vi "Activate dub.vi"(7 "DO Task":refnum<k21>, 8 "error constant":errorcluster, 11 "DO":T1(array[cluster])=[{"CDT"=-150.0, "Position"=TRUE, "Component ID"="F_EPV_131"}, {"CDT"=-150.0, "Position"=TRUE, "Component ID"="F_EPV_131"}, {"CDT"=-135.0, "Position"=FALSE, "Component ID"="F_EPV_132"}, {"CDT"=-120.0, "Position"=FALSE, "Component ID"="F_EPV_131"}, {"CDT"=-20.0, "Position"=TRUE, "Component ID"="F_EPV_136"}, {"CDT"=-10.0, "Position"=FALSE, "Component ID"="F_EPV_136"}]) -> (0 "error out":errorcluster, 3 "Abort":bool)   [LabVIEW 2022 SP3]
uses:
  RT Controls/DO FGV.ctl
  <vilib>/DAQmx/write.llb/DAQmx Write (Digital 1D Bool NChan 1Samp 1Line).vi
  RT Sub VI's/RT Global.vi
  <vilib>/DAQmx/miscellaneous.llb/DAQmx Fill In Error Info.vi
panel:
  out "Launch Time":timestamp
  out "DO value":bool[](array[boolean])
  out "Status":string
  out "x-y":dbl
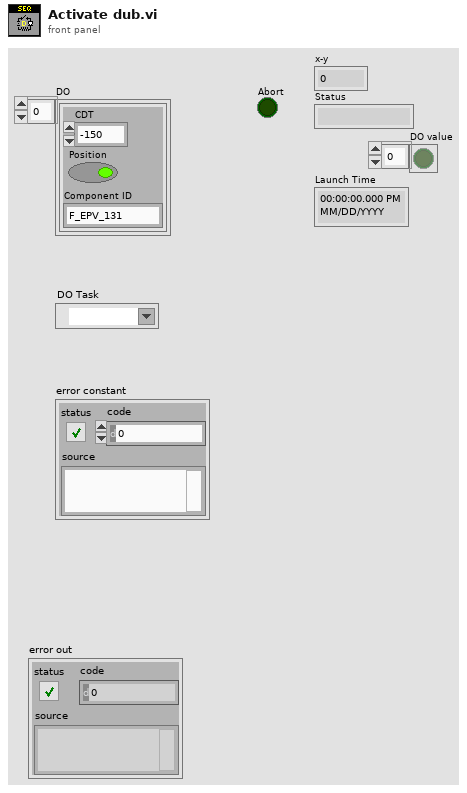
[diagram p1: front panel]
types:
  T1 = cluster{"CDT":dbl, "Position":bool, "Component ID":string}[]
  T2 = cluster{"AO":cluster{"CDT":dbl, "Range":dbl, "Component ID":string}[], "DO":cluster{"CDT":dbl, "Position":bool, "Component ID":string}[], "Launch Time":timestamp}
  T3 = typedef "DO FGV.ctl" = enum16{"Read", "Write", "Start time", "init", "Read only"}
  T4 = cluster{"CDT":dbl, "Position":bool, "Component ID":string}
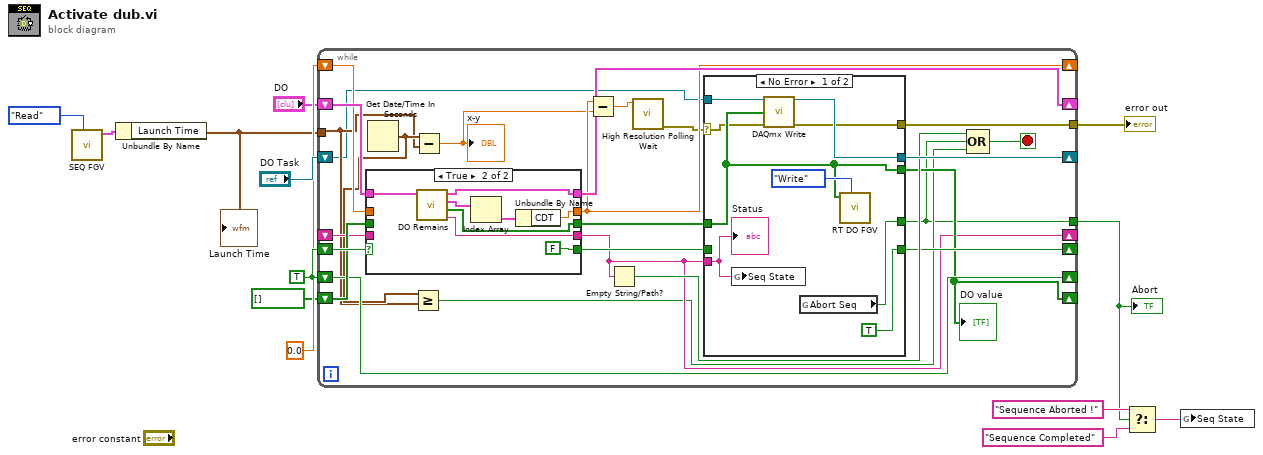
[diagram p0: block diagram]
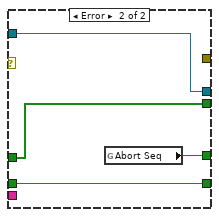
[diagram p2: hidden frame]
diagram:
  w13 = TRUE
  n1 = call "SEQ FGV.vi"("Enum"=enum16{"Read", "Write"}."Read") -> ("Seq data out"=w10:T2)  [unwired: 9 in, 1 out]
  n2 = Unbundle By Name(w10) -> ("Launch Time"=w1:timestamp)
  "Launch Time" <- w1
  n3 = while {
    shift-right: [w30] -> _
    shift-left: "DO" -> [w38]
    shift-right: [w27] -> _
    shift-left: w13 -> [w37]
    shift-right: [w26] -> _
    shift-left: bool[] [] ("DO value") -> [w36]
    shift-right: [w20] -> _
    shift-left: 0.0 ("CDT") -> [w35]
    shift-right: [w33] -> _
    shift-left: w13 -> [w33]
    shift-right: [w32] -> _
    shift-left: "DO Task" -> [w15]
    tunnel: [w16] -> w4
    tunnel: w1 -> [w22]
    shift-right: [w24] -> _
    shift-left: _ -> [w25]
    tunnel: [w17] -> w3
    stop <- w31 stop-if-true
    n4 = case shown="True" w37 {
      selector: w37 -> [w53 _]
      tunnel: w38 -> [w54 w64]
      tunnel: [w54 w59] -> w30
      tunnel: [w56 w61] -> w34
      tunnel: w36 -> [w56 _]
      tunnel: [w55 w60] -> w20
      tunnel: w35 -> [w55 _]
      tunnel: [w53 FALSE] -> w28
      tunnel: [w52 w57] -> w24
      tunnel: w25 -> [w52 _]
      frame False {
      }
      frame True {
        n5 = call "DO Remains.vi"("Array"=w64) -> ("Status"=w57:string, "DO value"=w61:bool[], "Same DO"=w63:T1, "Remains"=w59:T1)  [unwired: 7 in]
        n6 = Index Array(array=w63) -> (element=w62:T4)  [unwired: 1 in]
        n7 = Unbundle By Name(w62) -> ("CDT"=w60:dbl)
      }
    }
    n8 = Get Date/Time In Seconds() -> (seconds since 1Jan1904=w23:timestamp)
    n9 = Greater Or Equal?(x=w23, y=w22) -> (x >= y?=w21:bool)
    n10 = Subtract(x=w23, y=w22) -> (x-y=w19:dbl)
    "x-y" <- w19
    n11 = Subtract(x=w20, y=w19) -> (x-y=w14:dbl)
    n12 = Empty String/Path?(string/path=w24) -> (empty?=w29:bool)
    n13 = call <vilib>:"High Resolution Polling Wait.vi"("seconds to wait"=w14) -> ("error out"=w18:errorcluster)  [unwired: 10 in]
    n14 = case shown="No Error" w18 {
      selector: w18 -> [w40 _]
      tunnel: w34 -> [w41 w51]
      tunnel: [w41 w51] -> w26
      tunnel: w15 -> [w47 w50]
      tunnel: [w46 w50] -> w32
      tunnel: [w45 _] -> w17
      tunnel: w28 -> [_ w49]
      tunnel: [TRUE w49] -> w27
      tunnel: w24 -> [w43 _]
      tunnel: [w39 w48] -> w16
      frame No Error {
        n15 = global write "RT Global.vi" "Seq State"(w43) -> ()
        n16 = call-poly <vilib>:"DAQmx Write.vi"("task/channels in"=w47, "data"=w41, "error in"=w40) -> ("task out"=w46:refnum<k21>, "error out"=w45:errorcluster)  [unwired: 10 in, 1 out]
        n17 = global read "RT Global.vi" "Abort Seq"() -> (w39:bool)
        n18 = call "RT DO FGV.vi"("Enum"=DO_FGV."Write", "DO in"=w41) -> ()  [unwired: 7 in, 3 out]
        "Status" <- w43
      }
      frame Error {
        n19 = global read "RT Global.vi" "Abort Seq"() -> (w48:bool)
      }
    }
    "DO value" <- w26
    n20 = Compound Arithmetic op=OR(w29, w16, w21) -> (w31:bool)
  }
  "Abort" <- w4
  "error out" <- w3
  n21 = Select(t="Sequence Aborted !" ("Seq State"), s=w4, f="Sequence Completed" ("Seq State")) -> (s? t:f=w5:string)
  n22 = global write "RT Global.vi" "Seq State"(w5) -> ()
